vi "LTrim.vi"(0 "reference in":refnum<class "Redis.lvclass">, 1 "Key":string, 5 "Start Index":i32, 9 "Stop Index":i32, 11 "Error In":errorcluster) -> (4 "reference out":refnum<class "Redis.lvclass">, 8 "Elements":string[](array[string]), 15 "Error Out":errorcluster)   [LabVIEW 2020, in "Redis.lvclass"]
doc: "<b>LTRIM</b>\n\nTrim an existing list so that it will contain only the specified range of elements specified. Both start and stop are zero-based indexes, where 0 is the first element of the list (the head), 1 the next element and so on.\n\nFor example: LTRIM foobar 0 2 will modify the list stored at foobar so that only the first three elements of the list will remain.\n\nstart and end can also be negative numbers indicating offsets from the end of the list, where -1 is the last element of the list, -2 the penultimate element and so on.\n\nOut of range indexes will not produce an error: if start is larger than the end of the list, or start > end, the result will be an empty list (which causes key to be removed). If end is larger than the end of the list, Redis will treat it like the last element of the list."
uses:
  Redis.lvclass
  Redis.lvclass/Redis.ctl
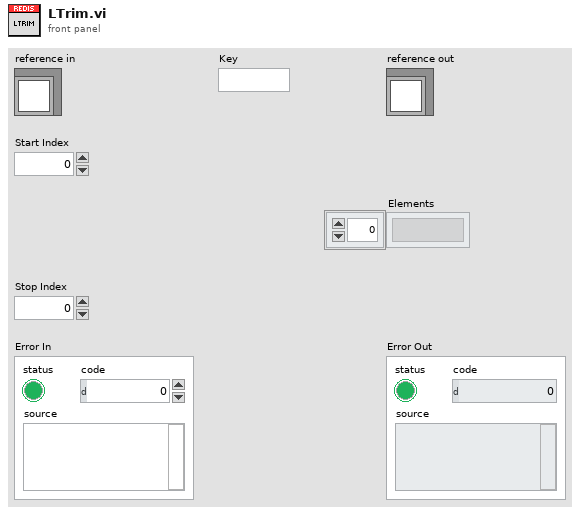
[diagram p1: front panel]
types:
  T1 = typedef "Redis.lvclass/RedisDataType.ctl" = cluster{"Reply Type":T2, "Integer":i64, "String":string, "Multibulk":variant[], "StringData":string[]}
  T2 = typedef "Redis.lvclass/ReplyDataTypeEnum.ctl" = enum16{"None", "Error", "Status", "Nil", "Integer", "String", "Multibulk"}
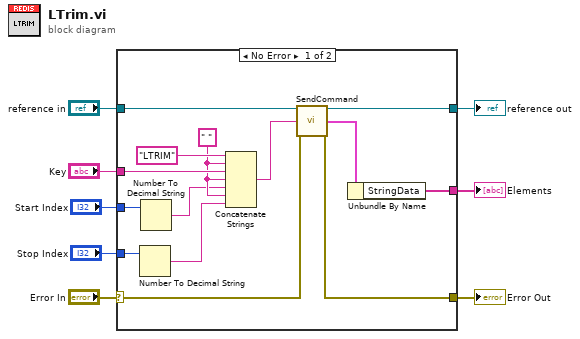
[diagram p0: block diagram]
diagram:
  n1 = case shown="No Error" "Error In" {
    selector: "Error In" -> [w20 w24]
    tunnel: [w10 w24] -> w7
    tunnel: [w22 w23] -> w5
    tunnel: "reference in" -> [w21 w23]
    tunnel: "Key" -> [w18 _]
    tunnel: "Start Index" -> [w15 _]
    tunnel: "Stop Index" -> [w14 _]
    tunnel: [w9 _] -> w1
    frame No Error {
      w13 = " "
      n2 = Number To Decimal String(number=w14) -> (decimal integer string=w11:string)  [unwired: 1 in]
      n3 = Number To Decimal String(number=w15) -> (decimal integer string=w12:string)  [unwired: 1 in]
      n4 = Concatenate Strings("LTRIM", w13, w18, w13, w12, w13, w11) -> (w17:string)
      n5 = call "SendCommand.vi"("reference in"=w21, "Command"=w17, "Error In"=w20) -> ("reference out"=w22:refnum<class "Redis.lvclass">, "Data"=w16:T1, "Error Out"=w10:errorcluster)  [unwired: 10 in]
      n6 = Unbundle By Name(w16) -> ("StringData"=w9:string[])
    }
    frame Error {
    }
  }
  "Error Out" <- w7
  "reference out" <- w5
  "Elements" <- w1
